vi "SensorReadAndWrite.vi"() -> ()   [LabVIEW 2023]
doc: "This VI shows how to setup and execute a measurement without any user input."
panel:
  out "Numeric":i32
  out "VI wird beendet":string
  in  "VI-Stopp":bool
  out "Diagram 2":waveform(dbl)(graph)
  in  "Kanal 2":i32=2 min=1 max=4 step=1
  in  "Kanal":i32=1 min=1 max=4 step=1
  in  "Datei-Pfad":path
  out "Diagram":waveform(dbl)(graph)
  in  "Messung":bool=TRUE
  out "HBM Driver\nLicense is valid":bool
  # "Datenaufzeichnung"
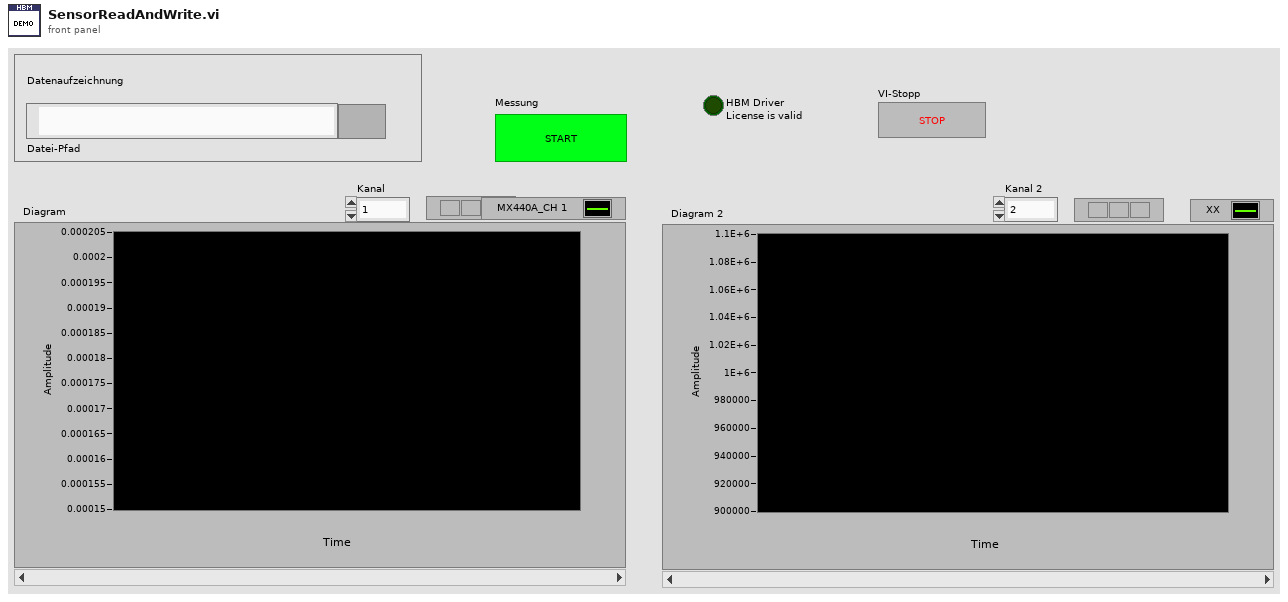
[diagram p1: front panel]
types:
  T1 = cluster{"Devices":refnum<k24>[], "Signals":refnum<k24>[]}
  T2 = enum16{"open", "replace", "create", "open or create", "replace or create", "replace or create with confirmation"}
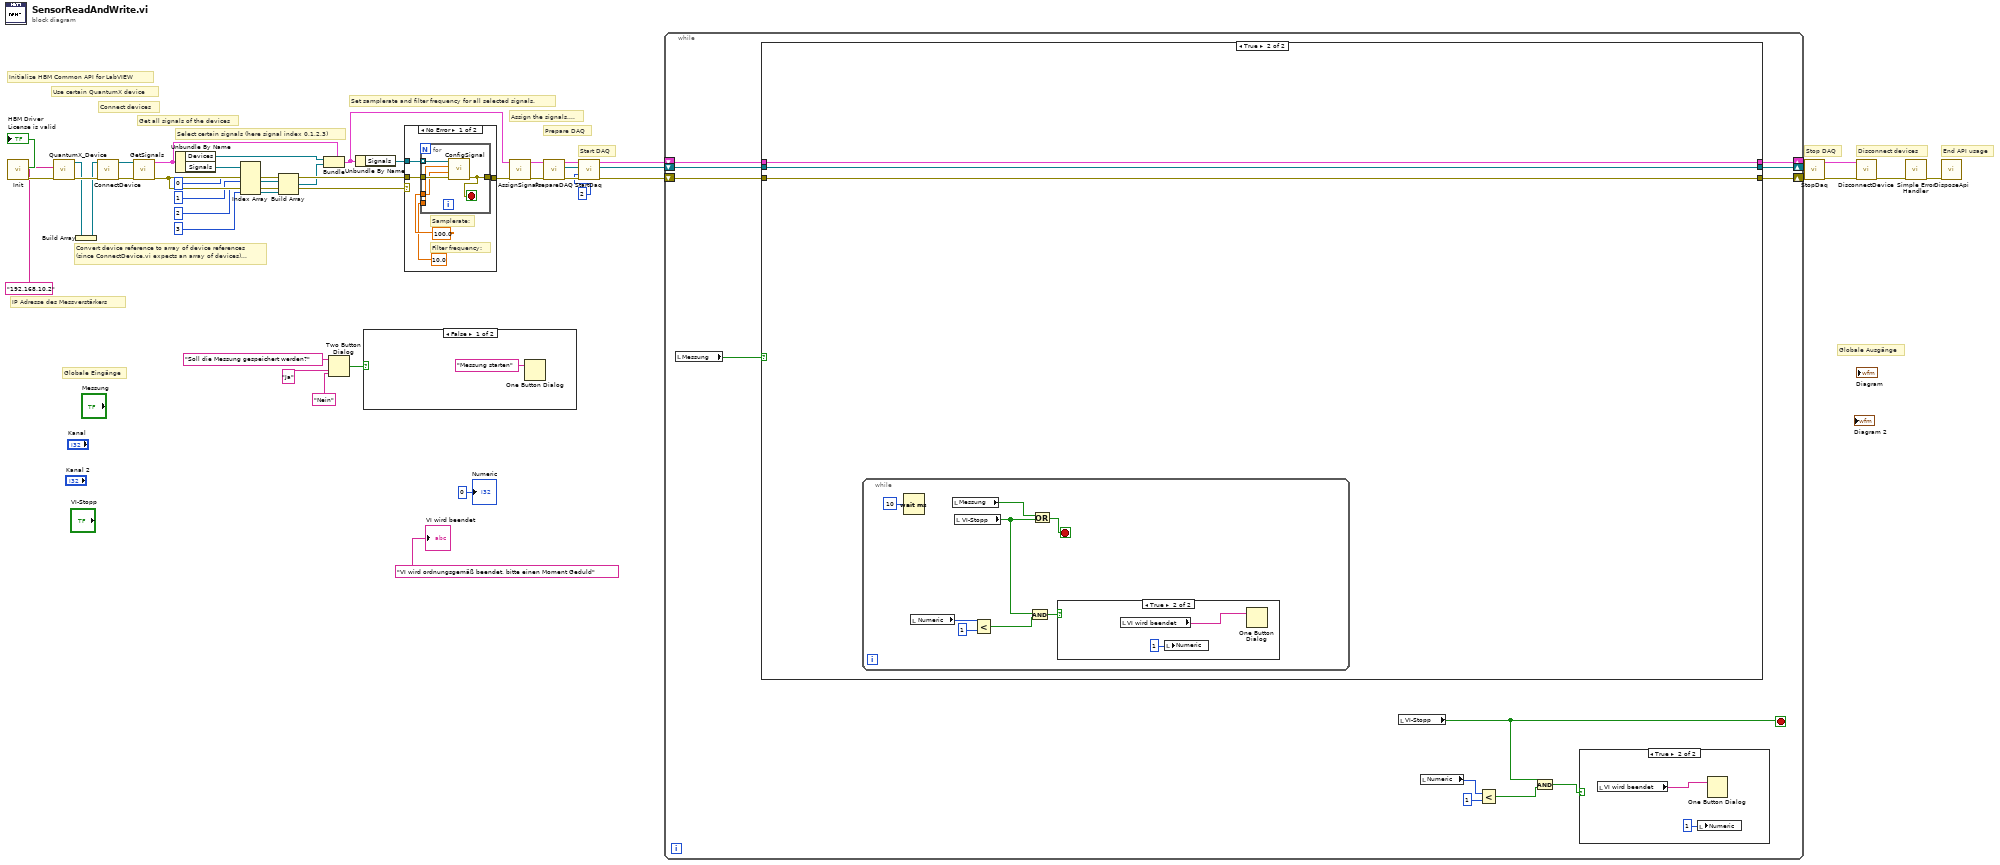
[diagram p0: block diagram]
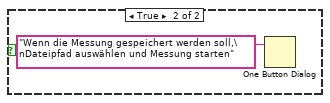
[diagram p2: hidden frame]
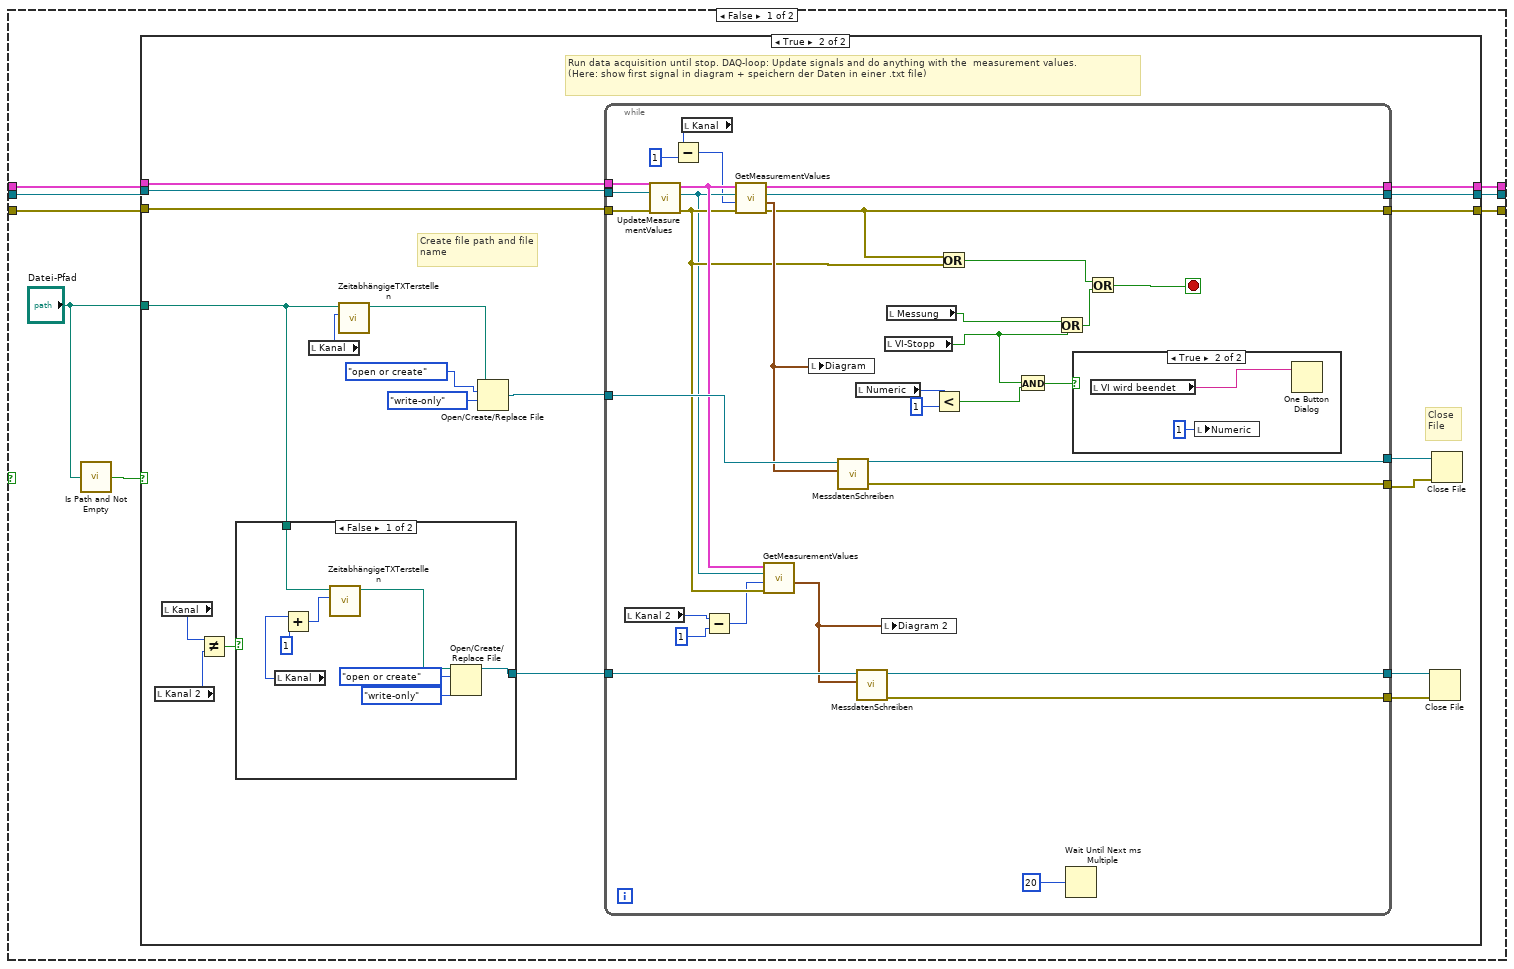
[diagram p4: hidden frame]
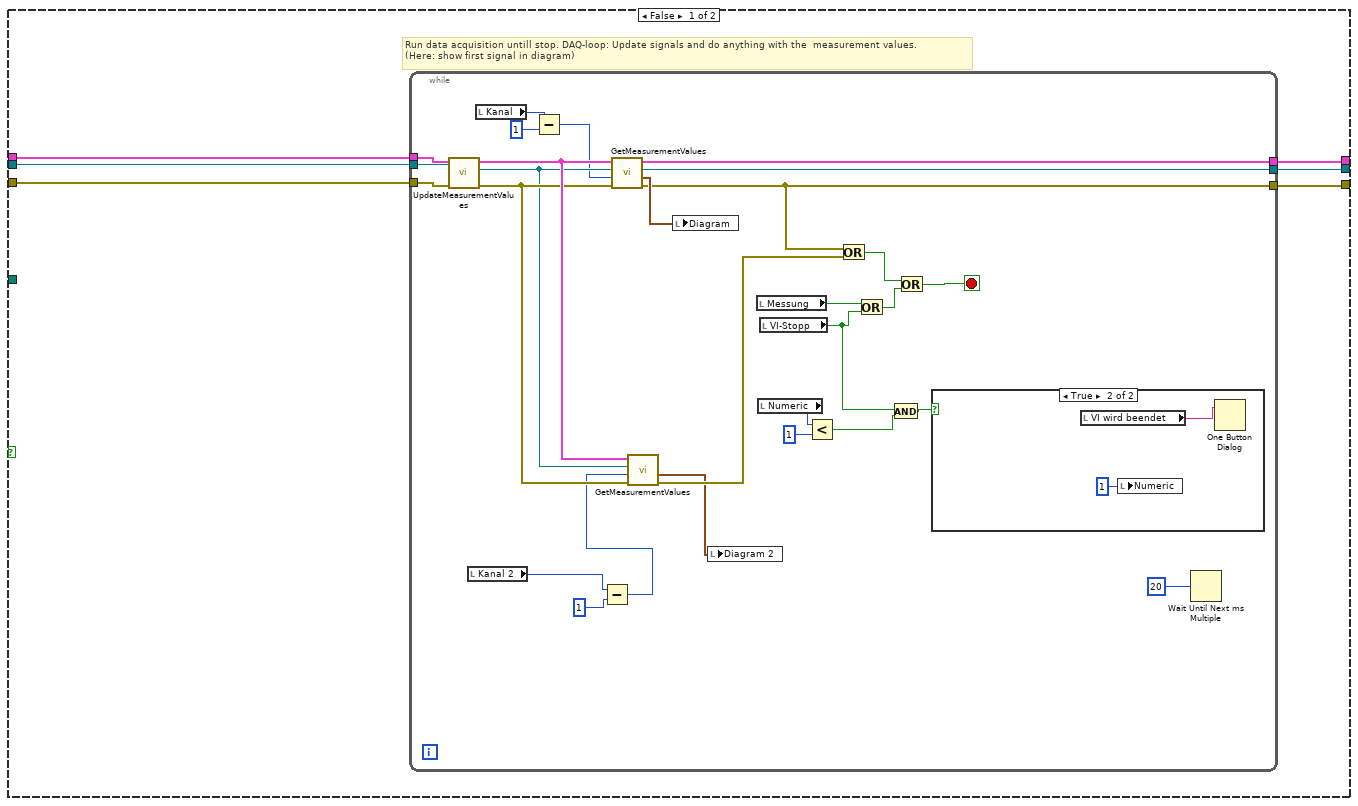
[diagram p5: hidden frame]
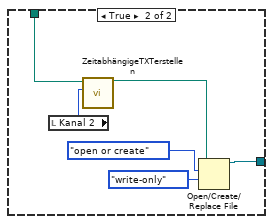
[diagram p7: hidden frame]
diagram:
  # "Globale Ausgänge"
  # "Globale Eingänge"
  # "IP Adresse des Messverstärkers"
  # "Convert device reference to array of device references\n(since ConnectDevice.vi expects an array of devices)..."
  # "Disconnect devices"
  # "Set samplerate and filter frequency for all selected signals."
  # "Initialize HBM Common API for LabVIEW"
  # "End API usage"
  # "Stop DAQ"
  # "Start DAQ"
  # "Prepare DAQ"
  # "Select certain signals (here signal index 0,1,2,3)"
  # "Get all signals of the devices"
  # "Connect devices"
  # "Use certain QuantumX device"
  # "Assign the signals...."
  n1 = call "Init.vi"() -> ("LicenseIsValid"=→"HBM Driver\nLicense is valid":bool, "Error out"=w16:errorcluster)  [unwired: 8 in, 1 out]
  n2 = call "QuantumX_Device.vi"("Error in"=w16, "IPAddress"="192.168.10.2" ("IPAddress of QuantumX device")) -> ("Error out"=w17:errorcluster, "Device"=w14:refnum<k24>)  [unwired: 6 in]
  n3 = Build Array(w14) -> (w13:refnum<k24>[])
  n4 = call "ConnectDevice.vi"("Error in"=w17, "Devices"=w13) -> ("Error out"=w39:errorcluster, "Devices"=w38:refnum<k24>[])  [unwired: 7 in, 1 out]
  n5 = call "GetSignals.vi"("Error in"=w39, "Devices"=w38) -> ("Error out"=w33:errorcluster, "DevicesAndSignals"=w34:T1)  [unwired: 8 in]
  n6 = Unbundle By Name(w34) -> ("Devices"=w27:refnum<k24>[], "Signals"=w31:refnum<k24>[])
  n7 = Index Array(array=w31, index #1=0 ("Index"), index #2=1 ("Index"), index #3=2 ("Index"), index #4=3 ("Index")) -> (element #1=w30:refnum<k24>, element #2=w29:refnum<k24>, element #3=w22:refnum<k24>, element #4=w21:refnum<k24>)
  n8 = Build Array(w30, w29, w22, w21) -> (w28:refnum<k24>[])
  n9 = Bundle(cluster=w34, "Devices"=w27, "Signals"=w28) -> (w35:T1)
  n10 = Two Button Dialog(message="Soll die Messung gespeichert werden?", 1:"Nein" ("F button name (\"Cancel\")"), 2:"Ja" ("T button name (\"OK\")")) -> (T button?=w6:bool)
  n11 = Unbundle By Name(w35) -> ("Signals"=w46:refnum<k24>[])
  n12 = case shown="False" w6 {
    frame False {
      n13 = One Button Dialog(message="Messung starten") -> ()  [unwired: 1 in, 1 out]
    }
    frame True {
      n14 = One Button Dialog(message="Wenn die Messung gespeichert werden soll,\nDateipfad auswählen und Messung starten") -> ()  [unwired: 1 in, 1 out]
    }
  }
  n15 = case shown="No Error" w33 {
    tunnel: w33 -> [w53 w59]
    tunnel: w46 -> [w52 _]
    tunnel: [w51 w59] -> w45
    frame No Error {
      # "Filter frequency:"
      # "Samplerate:"
      n16 = for {
        tunnel: w53 -> [w58]
        tunnel: 100.0 ("SampleRate") -> [w57]
        tunnel: 10.0 ("FilterFrequency") -> [w56]
        tunnel: w52 -> [w55] mode=indexing
        tunnel: [w54] -> w51
        stop <- w54 stop-if-true
        n17 = call "ConfigSignal.vi"("Error in"=w58, "SampleRate"=w57, "FilterFrequency"=w56, "Signal"=w55) -> ("Error out"=w54:errorcluster)  [unwired: 7 in]
      }
    }
    frame Error {
    }
  }
  n18 = call "AssignSignals.vi"("Error in"=w45, "DevicesAndSignals"=w35) -> ("Error out"=w43:errorcluster, "DevicesAndSignals"=w44:T1)  [unwired: 8 in]
  n19 = call "PrepareDAQ.vi"("Error in"=w43, "DevicesAndSignals"=w44) -> ("Error out"=w40:errorcluster, "DaqMeasurement"=w41:refnum<k24>, "DevicesAndSignals"=w42:T1)  [unwired: 7 in]
  n20 = call "StartDaq.vi"("DevicesAndSignals"=w42, "DaqMeasurement"=w41, "AcquisitionMode"=2, "Error in"=w40) -> ("DevicesAndSignals"=w9:T1, "DaqMeasurement"=w8:refnum<k24>, "Error out"=w7:errorcluster)  [unwired: 7 in, 2 out]
  n21 = while {
    shift-right: [w71] -> w11
    shift-left: w9 -> [w69]
    shift-right: [w65] -> w12
    shift-left: w8 -> [w68]
    shift-right: [w70] -> w10
    shift-left: w7 -> [w67]
    stop <- w61 stop-if-true
    n22 = local read "Messung"() -> (w66:bool)
    n23 = case shown="True" w66 {
      tunnel: [w80 w189] -> w71
      tunnel: [w79 w187] -> w70
      tunnel: w69 -> [w78 w189]
      tunnel: w68 -> [w77 w188]
      tunnel: w67 -> [w76 w187]
      tunnel: [w81 w188] -> w65
      frame False {
        n24 = call <vilib>:"Is Path and Not Empty.vi"("path"="Datei-Pfad") -> ("Is Path and Not Empty?"=w74:bool)  [unwired: 4 in]
        n25 = case shown="True" w74 {
          tunnel: [w83 w135] -> w81
          tunnel: [w84 w134] -> w80
          tunnel: [w82 w133] -> w79
          tunnel: w78 -> [w87 w132]
          tunnel: w77 -> [w86 w131]
          tunnel: w76 -> [w85 w130]
          tunnel: "Datei-Pfad" -> [_ w126]
          frame False {
            # "Run data acquisition untill stop. DAQ-loop: Update signals and do anything with the  measurement values.\n(Here: show first signal in diagram)"
            n26 = while {
              tunnel: [w115] -> w83
              tunnel: [w114] -> w84
              tunnel: [w107] -> w82
              tunnel: w87 -> [w112]
              tunnel: w86 -> [w111]
              tunnel: w85 -> [w110]
              stop <- w93 stop-if-true
              n27 = call "UpdateMeasurementValues.vi"("Error in"=w110, "DaqMeasurement"=w111, "DevicesAndSignals"=w112) -> ("Error out"=w105:errorcluster, "DaqMeasurement"=w104:refnum<k24>, "DevicesAndSignals"=w106:T1)  [unwired: 6 in]
              n28 = local read "Kanal 2"() -> (w97:i32)
              n29 = local read "Kanal"() -> (w100:i32)
              n30 = Subtract(x=w100, y=1) -> (x-y=w99:i32)
              n31 = Subtract(x=w97, y=1) -> (x-y=w96:i32)
              n32 = call "GetMeasurementValues.vi"("Error in"=w105, "Index"=w99, "DaqMeasurement"=w104, "DevicesAndSignals"=w106) -> ("Error out"=w107:errorcluster, "Waveform"=w109:waveform(dbl), "DaqMeasurement"=w115:refnum<k24>, "DevicesAndSignals"=w114:T1)  [unwired: 2 in, 2 out]
              n33 = call "GetMeasurementValues.vi"("Error in"=w105, "Index"=w96, "DaqMeasurement"=w104, "DevicesAndSignals"=w106) -> ("Error out"=w103:errorcluster, "Waveform"=w102:waveform(dbl))  [unwired: 2 in, 4 out]
              n34 = local write "Diagram"(w109) -> ()
              n35 = local write "Diagram 2"(w102) -> ()
              n36 = local read "Messung"() -> (w94:bool)
              n37 = local read "Numeric"() -> (w88:i32)
              n38 = local read "VI-Stopp"() -> (w90:bool)
              n39 = Less?(x=w88, y=1) -> (x < y?=w91:bool)
              n40 = Or(x=w107, y=w103) -> (x .or. y?=w108:bool)
              n41 = Or(x=w94, y=w90) -> (x .or. y?=w95:bool)
              n42 = And(x=w90, y=w91) -> (x .and. y?=w89:bool)
              n43 = Or(x=w108, y=w95) -> (x .or. y?=w93:bool)
              n44 = case shown="True" w89 {
                frame False {
                }
                frame True {
                  n45 = local read "VI wird beendet"() -> (w117:string)
                  n46 = local write "Numeric"(1 ("Numeric")) -> ()
                  n47 = One Button Dialog(message=w117) -> ()  [unwired: 1 in, 1 out]
                }
              }
              n48 = Wait Until Next ms Multiple(millisecond multiple=u32 20 ("Vielfache von ms")) -> ()  [unwired: 1 out]
            }
          }
          frame True {
            # "Close\nFile"
            # "Create file path and file name"
            # "Run data acquisition until stop. DAQ-loop: Update signals and do anything with the  measurement values.\n(Here: show first signal in diagram + speichern der Daten in einer .txt file)"
            n49 = local read "Kanal 2"() -> (w118:i32)
            n50 = local read "Kanal"() -> (w119:i32)
            n51 = Not Equal?(x=w119, y=w118) -> (x != y?=w120:bool)
            n52 = case shown="False" w120 {
              tunnel: w126 -> [w145 w149]
              tunnel: [w141 w146] -> w123
              frame False {
                n53 = local read "Kanal"() -> (w143:i32)
                n54 = Add(x=w143, y=1) -> (x+y=w144:i32)
                n55 = call "ZeitabhängigeTXTerstellen.vi"("Signal index to display"=w144, "path"=w145) -> ("Path"=w140:path)  [unwired: 9 in]
                n56 = Open/Create/Replace File(file path (use dialog)=w140, operation (0:open)=T2."open or create", access (0:read/write)=enum16{"read/write", "read-only", "write-only"}."write-only") -> (refnum out=w141:refnum<file>)  [unwired: 3 in, 2 out]
              }
              frame True {
                n57 = local read "Kanal 2"() -> (w151:i32)
                n58 = call "ZeitabhängigeTXTerstellen.vi"("Signal index to display"=w151, "path"=w149) -> ("Path"=w150:path)  [unwired: 9 in]
                n59 = Open/Create/Replace File(file path (use dialog)=w150, operation (0:open)=T2."open or create", access (0:read/write)=enum16{"read/write", "read-only", "write-only"}."write-only") -> (refnum out=w146:refnum<file>)  [unwired: 3 in, 2 out]
              }
            }
            n60 = local read "Kanal"() -> (w127:i32)
            n61 = call "ZeitabhängigeTXTerstellen.vi"("Signal index to display"=w127, "path"=w126) -> ("Path"=w121:path)  [unwired: 9 in]
            n62 = Open/Create/Replace File(file path (use dialog)=w121, operation (0:open)=T2."open or create", access (0:read/write)=enum16{"read/write", "read-only", "write-only"}."write-only") -> (refnum out=w122:refnum<file>)  [unwired: 3 in, 2 out]
            n63 = while {
              tunnel: w131 -> [w183]
              tunnel: [w182] -> w135
              tunnel: [w181] -> w134
              tunnel: w130 -> [w184]
              tunnel: [w168] -> w133
              tunnel: [w178] -> w137
              tunnel: [w177] -> w136
              tunnel: w122 -> [w176]
              tunnel: w132 -> [w175]
              tunnel: w123 -> [w170]
              tunnel: [w173] -> w129
              tunnel: [w172] -> w128
              stop <- w179 stop-if-true
              n64 = local read "Kanal 2"() -> (w160:i32)
              n65 = call "UpdateMeasurementValues.vi"("Error in"=w184, "DaqMeasurement"=w183, "DevicesAndSignals"=w175) -> ("Error out"=w167:errorcluster, "DaqMeasurement"=w165:refnum<k24>, "DevicesAndSignals"=w171:T1)  [unwired: 6 in]
              n66 = local read "Kanal"() -> (w164:i32)
              n67 = Subtract(x=w164, y=1) -> (x-y=w162:i32)
              n68 = Subtract(x=w160, y=1) -> (x-y=w159:i32)
              n69 = call "GetMeasurementValues.vi"("Error in"=w167, "Index"=w162, "DaqMeasurement"=w165, "DevicesAndSignals"=w171) -> ("Error out"=w168:errorcluster, "Waveform"=w174:waveform(dbl), "DaqMeasurement"=w182:refnum<k24>, "DevicesAndSignals"=w181:T1)  [unwired: 2 in, 2 out]
              n70 = call "GetMeasurementValues.vi"("Error in"=w167, "Index"=w159, "DaqMeasurement"=w165, "DevicesAndSignals"=w171) -> ("Waveform"=w169:waveform(dbl))  [unwired: 2 in, 5 out]
              n71 = local write "Diagram"(w174) -> ()
              n72 = call "MessdatenSchreiben.vi"("Waveform"=w174, "Byte Stream File in"=w176) -> ("error out"=w178:errorcluster, "Byte Stream File out"=w177:refnum<file>)  [unwired: 8 in]
              n73 = local read "Numeric"() -> (w152:i32)
              n74 = call "MessdatenSchreiben.vi"("Waveform"=w169, "Byte Stream File in"=w170) -> ("error out"=w172:errorcluster, "Byte Stream File out"=w173:refnum<file>)  [unwired: 8 in]
              n75 = local write "Diagram 2"(w169) -> ()
              n76 = local read "VI-Stopp"() -> (w154:bool)
              n77 = local read "Messung"() -> (w157:bool)
              n78 = Less?(x=w152, y=1) -> (x < y?=w155:bool)
              n79 = Or(x=w168, y=w167) -> (x .or. y?=w166:bool)
              n80 = And(x=w154, y=w155) -> (x .and. y?=w153:bool)
              n81 = Or(x=w157, y=w154) -> (x .or. y?=w158:bool)
              n82 = Wait Until Next ms Multiple(millisecond multiple=u32 20 ("Vielfache von ms")) -> ()  [unwired: 1 out]
              n83 = case shown="True" w153 {
                frame False {
                }
                frame True {
                  n84 = local read "VI wird beendet"() -> (w186:string)
                  n85 = local write "Numeric"(1 ("Numeric")) -> ()
                  n86 = One Button Dialog(message=w186) -> ()  [unwired: 1 in, 1 out]
                }
              }
              n87 = Or(x=w166, y=w158) -> (x .or. y?=w179:bool)
            }
            n88 = Close File(refnum=w129, error in=w128) -> ()  [unwired: 2 out]
            n89 = Close File(refnum=w136, error in=w137) -> ()  [unwired: 2 out]
          }
        }
      }
      frame True {
        n90 = while {
          stop <- w195 stop-if-true
          n91 = Wait (ms)(milliseconds to wait=u32 10) -> ()  [unwired: 1 out]
          n92 = local read "Numeric"() -> (w192:i32)
          n93 = local read "Messung"() -> (w196:bool)
          n94 = local read "VI-Stopp"() -> (w193:bool)
          n95 = Less?(x=w192, y=1) -> (x < y?=w190:bool)
          n96 = And(x=w193, y=w190) -> (x .and. y?=w194:bool)
          n97 = Or(x=w196, y=w193) -> (x .or. y?=w195:bool)
          n98 = case shown="True" w194 {
            frame False {
            }
            frame True {
              n99 = local read "VI wird beendet"() -> (w199:string)
              n100 = local write "Numeric"(1 ("Numeric")) -> ()
              n101 = One Button Dialog(message=w199) -> ()  [unwired: 1 in, 1 out]
            }
          }
        }
      }
    }
    n102 = local read "VI-Stopp"() -> (w61:bool)
    n103 = local read "Numeric"() -> (w60:i32)
    n104 = Less?(x=w60, y=1) -> (x < y?=w64:bool)
    n105 = And(x=w61, y=w64) -> (x .and. y?=w62:bool)
    n106 = case shown="True" w62 {
      frame False {
      }
      frame True {
        n107 = local read "VI wird beendet"() -> (w73:string)
        n108 = local write "Numeric"(1 ("Numeric")) -> ()
        n109 = One Button Dialog(message=w73) -> ()  [unwired: 1 in, 1 out]
      }
    }
  }
  n110 = call "StopDaq.vi"("Error in"=w10, "DaqMeasurement"=w12, "DevicesAndSignals"=w11) -> ("Error out"=w20:errorcluster, "DevicesAndSignals"=w19:T1)  [unwired: 7 in]
  n111 = call "DisconnectDevice.vi"("Error in"=w20, "DevicesAndSignals"=w19) -> ("Error out"=w18:errorcluster)  [unwired: 9 in]
  n112 = call <vilib>:"Simple Error Handler.vi"("error in (no error)"=w18) -> ("error out"=w37:errorcluster)  [unwired: 4 in, 4 out]
  n113 = call "DisposeApi.vi"("Error in"=w37) -> ()  [unwired: 10 in, 1 out]
  "VI wird beendet" <- "VI wird ordnungsgemäß beendet, bitte einen Moment Geduld"
  "Numeric" <- 0
